vi "Region Select.vi"(8 "Error In":errorcluster, 11 "Sensor Data Array":dbl[][](array[numeric])) -> (0 "Error Out":errorcluster, 1 "Trimmed Event":dbl[][](array[numeric]), 3 "Segement Start":dbl format="%.2f")   [LabVIEW 2020]
uses:
  <vilib>/Utility/miscctls.llb/LVCursorListTypeDef.ctl
panel:
  in  "Done":bool
  out "Sensor Plot":dbl[][](graph)
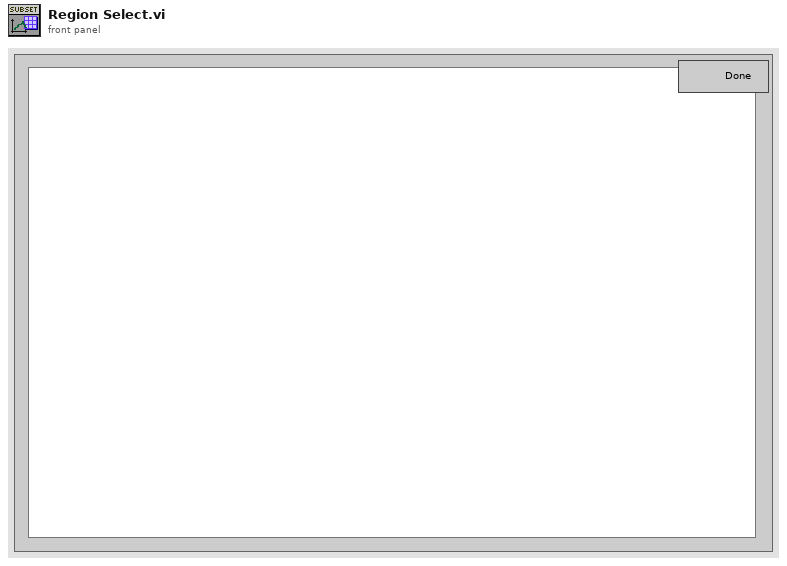
[diagram p1: front panel]
types:
  T1 = typedef "LVCursorListTypeDef.ctl" = cluster{"Name":string, "Color":u32, "Style":u8, "Point Style":u8, "Name Visible":bool, "Allow Drag":bool, "Cursor Mode":u32, "Plot":i32, "Index":i32, "Position":cluster{"X":dbl, "Y":dbl}, "X Scale":u32, "Y Scale":u32, "Watch Plots":i32[], "Watch All Plots":bool, "Plot Area":i32, "Label Offset":cluster{"X":dbl, "Y":dbl}}[]
  T2 = cluster{"Cursor List Cluster Constant Out[0]":cluster{"Name":string, "Color":u32, "Style":u8, "Point Style":u8, "Name Visible":bool, "Allow Drag":bool, "Cursor Mode":u32, "Plot":i32, "Index":i32, "Position":cluster{"X":dbl, "Y":dbl}, "X Scale":u32, "Y Scale":u32, "Watch Plots":i32[], "Watch All Plots":bool, "Plot Area":i32, "Label Offset":cluster{"X":dbl, "Y":dbl}}, "Cursor List Cluster Constant Out[1]":cluster{"Name":string, "Color":u32, "Style":u8, "Point Style":u8, "Name Visible":bool, "Allow Drag":bool, "Cursor Mode":u32, "Plot":i32, "Index":i32, "Position":cluster{"X":dbl, "Y":dbl}, "X Scale":u32, "Y Scale":u32, "Watch Plots":i32[], "Watch All Plots":bool, "Plot Area":i32, "Label Offset":cluster{"X":dbl, "Y":dbl}}, "Cursor List Cluster Constant Out[2]":cluster{"Name":string, "Color":u32, "Style":u8, "Point Style":u8, "Name Visible":bool, "Allow Drag":bool, "Cursor Mode":u32, "Plot":i32, "Index":i32, "Position":cluster{"X":dbl, "Y":dbl}, "X Scale":u32, "Y Scale":u32, "Watch Plots":i32[], "Watch All Plots":bool, "Plot Area":i32, "Label Offset":cluster{"X":dbl, "Y":dbl}}, "Cursor List Cluster Constant Out[3]":cluster{"Name":string, "Color":u32, "Style":u8, "Point Style":u8, "Name Visible":bool, "Allow Drag":bool, "Cursor Mode":u32, "Plot":i32, "Index":i32, "Position":cluster{"X":dbl, "Y":dbl}, "X Scale":u32, "Y Scale":u32, "Watch Plots":i32[], "Watch All Plots":bool, "Plot Area":i32, "Label Offset":cluster{"X":dbl, "Y":dbl}}, "Cursor List Cluster Constant Out[4]":cluster{"Name":string, "Color":u32, "Style":u8, "Point Style":u8, "Name Visible":bool, "Allow Drag":bool, "Cursor Mode":u32, "Plot":i32, "Index":i32, "Position":cluster{"X":dbl, "Y":dbl}, "X Scale":u32, "Y Scale":u32, "Watch Plots":i32[], "Watch All Plots":bool, "Plot Area":i32, "Label Offset":cluster{"X":dbl, "Y":dbl}}, "Cursor List Cluster Constant Out[5]":cluster{"Name":string, "Color":u32, "Style":u8, "Point Style":u8, "Name Visible":bool, "Allow Drag":bool, "Cursor Mode":u32, "Plot":i32, "Index":i32, "Position":cluster{"X":dbl, "Y":dbl}, "X Scale":u32, "Y Scale":u32, "Watch Plots":i32[], "Watch All Plots":bool, "Plot Area":i32, "Label Offset":cluster{"X":dbl, "Y":dbl}}, "Cursor List Cluster Constant Out[6]":cluster{"Name":string, "Color":u32, "Style":u8, "Point Style":u8, "Name Visible":bool, "Allow Drag":bool, "Cursor Mode":u32, "Plot":i32, "Index":i32, "Position":cluster{"X":dbl, "Y":dbl}, "X Scale":u32, "Y Scale":u32, "Watch Plots":i32[], "Watch All Plots":bool, "Plot Area":i32, "Label Offset":cluster{"X":dbl, "Y":dbl}}, "Cursor List Cluster Constant Out[7]":cluster{"Name":string, "Color":u32, "Style":u8, "Point Style":u8, "Name Visible":bool, "Allow Drag":bool, "Cursor Mode":u32, "Plot":i32, "Index":i32, "Position":cluster{"X":dbl, "Y":dbl}, "X Scale":u32, "Y Scale":u32, "Watch Plots":i32[], "Watch All Plots":bool, "Plot Area":i32, "Label Offset":cluster{"X":dbl, "Y":dbl}}, "Cursor List Cluster Constant Out[8]":cluster{"Name":string, "Color":u32, "Style":u8, "Point Style":u8, "Name Visible":bool, "Allow Drag":bool, "Cursor Mode":u32, "Plot":i32, "Index":i32, "Position":cluster{"X":dbl, "Y":dbl}, "X Scale":u32, "Y Scale":u32, "Watch Plots":i32[], "Watch All Plots":bool, "Plot Area":i32, "Label Offset":cluster{"X":dbl, "Y":dbl}}}
  T3 = cluster{"Name":string, "Color":u32, "Style":u8, "Point Style":u8, "Name Visible":bool, "Allow Drag":bool, "Cursor Mode":u32, "Plot":i32, "Index":i32, "Position":cluster{"X":dbl, "Y":dbl}, "X Scale":u32, "Y Scale":u32, "Watch Plots":i32[], "Watch All Plots":bool, "Plot Area":i32, "Label Offset":cluster{"X":dbl, "Y":dbl}}[]
  T4 = cluster{"CrsrList[0]":cluster{"Name":string, "Color":u32, "Style":u8, "Point Style":u8, "Name Visible":bool, "Allow Drag":bool, "Cursor Mode":u32, "Plot":i32, "Index":i32, "Position":cluster{"X":dbl, "Y":dbl}, "X Scale":u32, "Y Scale":u32, "Watch Plots":i32[], "Watch All Plots":bool, "Plot Area":i32, "Label Offset":cluster{"X":dbl, "Y":dbl}}, "CrsrList[1]":cluster{"Name":string, "Color":u32, "Style":u8, "Point Style":u8, "Name Visible":bool, "Allow Drag":bool, "Cursor Mode":u32, "Plot":i32, "Index":i32, "Position":cluster{"X":dbl, "Y":dbl}, "X Scale":u32, "Y Scale":u32, "Watch Plots":i32[], "Watch All Plots":bool, "Plot Area":i32, "Label Offset":cluster{"X":dbl, "Y":dbl}}, "CrsrList[2]":cluster{"Name":string, "Color":u32, "Style":u8, "Point Style":u8, "Name Visible":bool, "Allow Drag":bool, "Cursor Mode":u32, "Plot":i32, "Index":i32, "Position":cluster{"X":dbl, "Y":dbl}, "X Scale":u32, "Y Scale":u32, "Watch Plots":i32[], "Watch All Plots":bool, "Plot Area":i32, "Label Offset":cluster{"X":dbl, "Y":dbl}}, "CrsrList[3]":cluster{"Name":string, "Color":u32, "Style":u8, "Point Style":u8, "Name Visible":bool, "Allow Drag":bool, "Cursor Mode":u32, "Plot":i32, "Index":i32, "Position":cluster{"X":dbl, "Y":dbl}, "X Scale":u32, "Y Scale":u32, "Watch Plots":i32[], "Watch All Plots":bool, "Plot Area":i32, "Label Offset":cluster{"X":dbl, "Y":dbl}}, "CrsrList[4]":cluster{"Name":string, "Color":u32, "Style":u8, "Point Style":u8, "Name Visible":bool, "Allow Drag":bool, "Cursor Mode":u32, "Plot":i32, "Index":i32, "Position":cluster{"X":dbl, "Y":dbl}, "X Scale":u32, "Y Scale":u32, "Watch Plots":i32[], "Watch All Plots":bool, "Plot Area":i32, "Label Offset":cluster{"X":dbl, "Y":dbl}}, "CrsrList[5]":cluster{"Name":string, "Color":u32, "Style":u8, "Point Style":u8, "Name Visible":bool, "Allow Drag":bool, "Cursor Mode":u32, "Plot":i32, "Index":i32, "Position":cluster{"X":dbl, "Y":dbl}, "X Scale":u32, "Y Scale":u32, "Watch Plots":i32[], "Watch All Plots":bool, "Plot Area":i32, "Label Offset":cluster{"X":dbl, "Y":dbl}}, "CrsrList[6]":cluster{"Name":string, "Color":u32, "Style":u8, "Point Style":u8, "Name Visible":bool, "Allow Drag":bool, "Cursor Mode":u32, "Plot":i32, "Index":i32, "Position":cluster{"X":dbl, "Y":dbl}, "X Scale":u32, "Y Scale":u32, "Watch Plots":i32[], "Watch All Plots":bool, "Plot Area":i32, "Label Offset":cluster{"X":dbl, "Y":dbl}}, "CrsrList[7]":cluster{"Name":string, "Color":u32, "Style":u8, "Point Style":u8, "Name Visible":bool, "Allow Drag":bool, "Cursor Mode":u32, "Plot":i32, "Index":i32, "Position":cluster{"X":dbl, "Y":dbl}, "X Scale":u32, "Y Scale":u32, "Watch Plots":i32[], "Watch All Plots":bool, "Plot Area":i32, "Label Offset":cluster{"X":dbl, "Y":dbl}}, "CrsrList[8]":cluster{"Name":string, "Color":u32, "Style":u8, "Point Style":u8, "Name Visible":bool, "Allow Drag":bool, "Cursor Mode":u32, "Plot":i32, "Index":i32, "Position":cluster{"X":dbl, "Y":dbl}, "X Scale":u32, "Y Scale":u32, "Watch Plots":i32[], "Watch All Plots":bool, "Plot Area":i32, "Label Offset":cluster{"X":dbl, "Y":dbl}}}
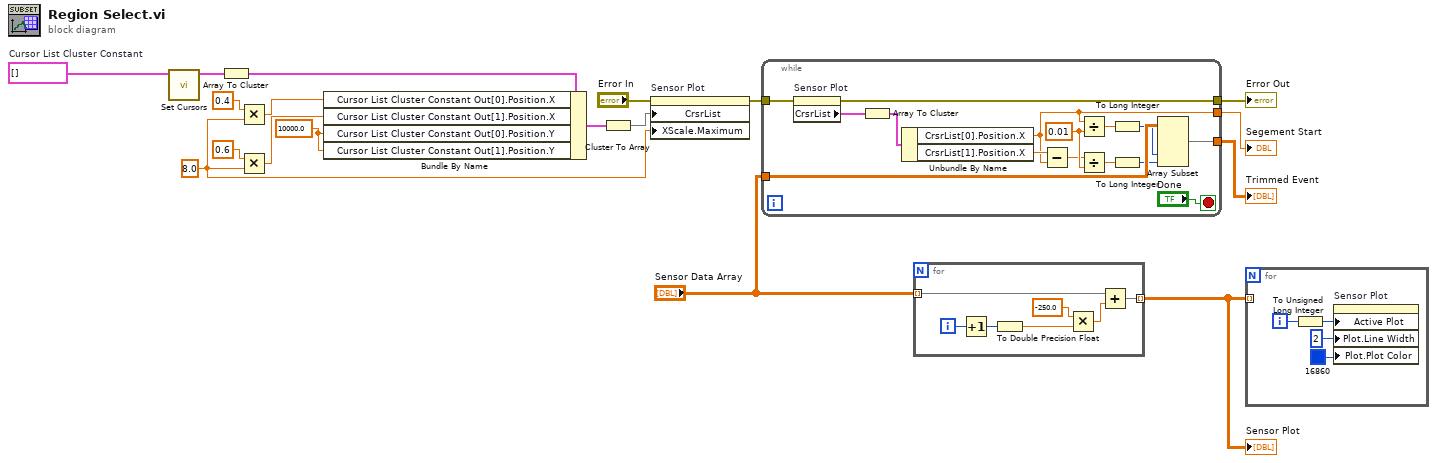
[diagram p0: block diagram]
diagram:
  w4 = 10000.0 ("Cursor List Cluster Constant Out[1].Position.Y")
  w7 = 8.0 ("X Scale.Range:Maximum")
  w16 = T1 []  # Cursor List Cluster Constant
  n1 = call "Set Cursors.vi"("Cursor List Cluster Constant in"=w16) -> ("Cursor List Cluster Constant Out"=w15:T1)  [unwired: 10 in]
  n2 = Array To Cluster(array=w15) -> (cluster=w14:T2)
  n3 = Multiply(x=0.4, y=w7) -> (x*y=w11:dbl)
  n4 = Multiply(x=0.6, y=w7) -> (x*y=w10:dbl)
  n5 = Bundle By Name(cluster=w14, "Cursor List Cluster Constant Out[0].Position.X"=w11, "Cursor List Cluster Constant Out[1].Position.X"=w10, "Cursor List Cluster Constant Out[0].Position.Y"=w4, "Cursor List Cluster Constant Out[1].Position.Y"=w4) -> (w13:T2)
  n6 = Cluster To Array(cluster=w13) -> (array=w12:T3)
  n7 = property on="Sensor Plot" class="WFGraph (strict)"(error in="Error In", "CrsrList"=w12, "XScale.Maximum"=w7) -> (error out=w6:errorcluster)  [unwired: 1 in, 1 out]
  n8 = while {
    tunnel: [w27] -> w18
    tunnel: "Sensor Data Array" -> [w26]
    tunnel: w6 -> [w25]
    tunnel: [w19] -> w5
    tunnel: [w23] -> w3
    stop <- "Done" stop-if-true
    w32 = 0.01 ("y")
    n9 = property on="Sensor Plot" class="WFGraph (strict)"(error in=w25) -> (error out=w27:errorcluster, "CrsrList"=w28:T1)  [unwired: 1 in, 1 out]
    n10 = Array To Cluster(array=w28) -> (cluster=w33:T4)
    n11 = Unbundle By Name(w33) -> ("CrsrList[0].Position.X"=w19:dbl, "CrsrList[1].Position.X"=w29:dbl)
    n12 = Subtract(x=w29, y=w19) -> (x-y=w30:dbl)
    n13 = Divide(x=w19, y=w32) -> (x/y=w20:dbl)
    n14 = Divide(x=w30, y=w32) -> (x/y=w31:dbl)
    n15 = To Long Integer(number=w20) -> (32bit integer=w22:i32)
    n16 = To Long Integer(number=w31) -> (32bit integer=w21:i32)
    n17 = Array Subset(array=w26, index (col)=w22, length (col)=w21) -> (w23:dbl[][])  [unwired: 2 in]
  }
  "Error Out" <- w18
  "Segement Start" <- w5
  "Trimmed Event" <- w3
  n18 = for {
    tunnel: "Sensor Data Array" -> [w40] mode=indexing
    tunnel: [w36] -> w1 mode=indexing
    i -> [w35]
    n19 = Increment(x=w35) -> (x+1=w34:i32)
    n20 = To Double Precision Float(number=w34) -> (double precision float=w39:dbl)
    n21 = Multiply(x=-250.0, y=w39) -> (x*y=w37:dbl)
    n22 = Add(x=w40, y=w37) -> (x+y=w36:dbl[])
  }
  "Sensor Plot" <- w1
  n23 = for {
    tunnel: w1 -> [_] mode=indexing
    i -> [w44]
    n24 = To Unsigned Long Integer(number=w44) -> (unsigned 32bit integer=w43:u32)
    n25 = property on="Sensor Plot" class="WFGraph (strict)"("Active Plot"=w43, "Plot.Line Width"=u8 2, "Plot.Plot Color"=u32 16860) -> ()  [unwired: 2 in, 2 out]
  }
